vi "Manuele override - backup voor overbelasting.vi"() -> ()   [LabVIEW 2019]
panel:
  out "richtingsaanwijzer":dbl(knob) scale=0.0..10.0
  in  "kruispunt":string
  out "bericht":string
  in  "STOP":bool
  in  "START":bool
  in  "stop 2":bool
  out "address":u32
  out "port":u16
  in  "stop":bool
  in  "vooruit":bool
  in  "achteruit":bool
  in  "links":bool
  in  "rechts":bool
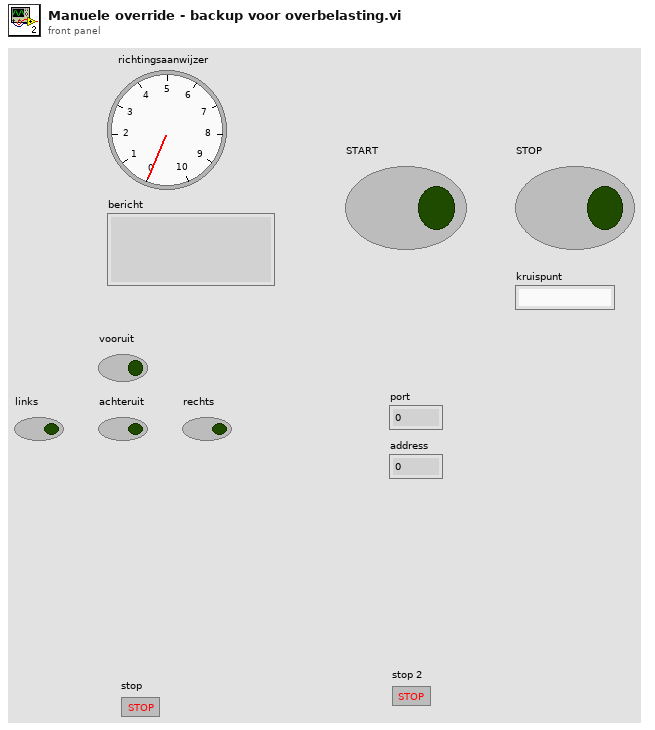
[diagram p1: front panel]
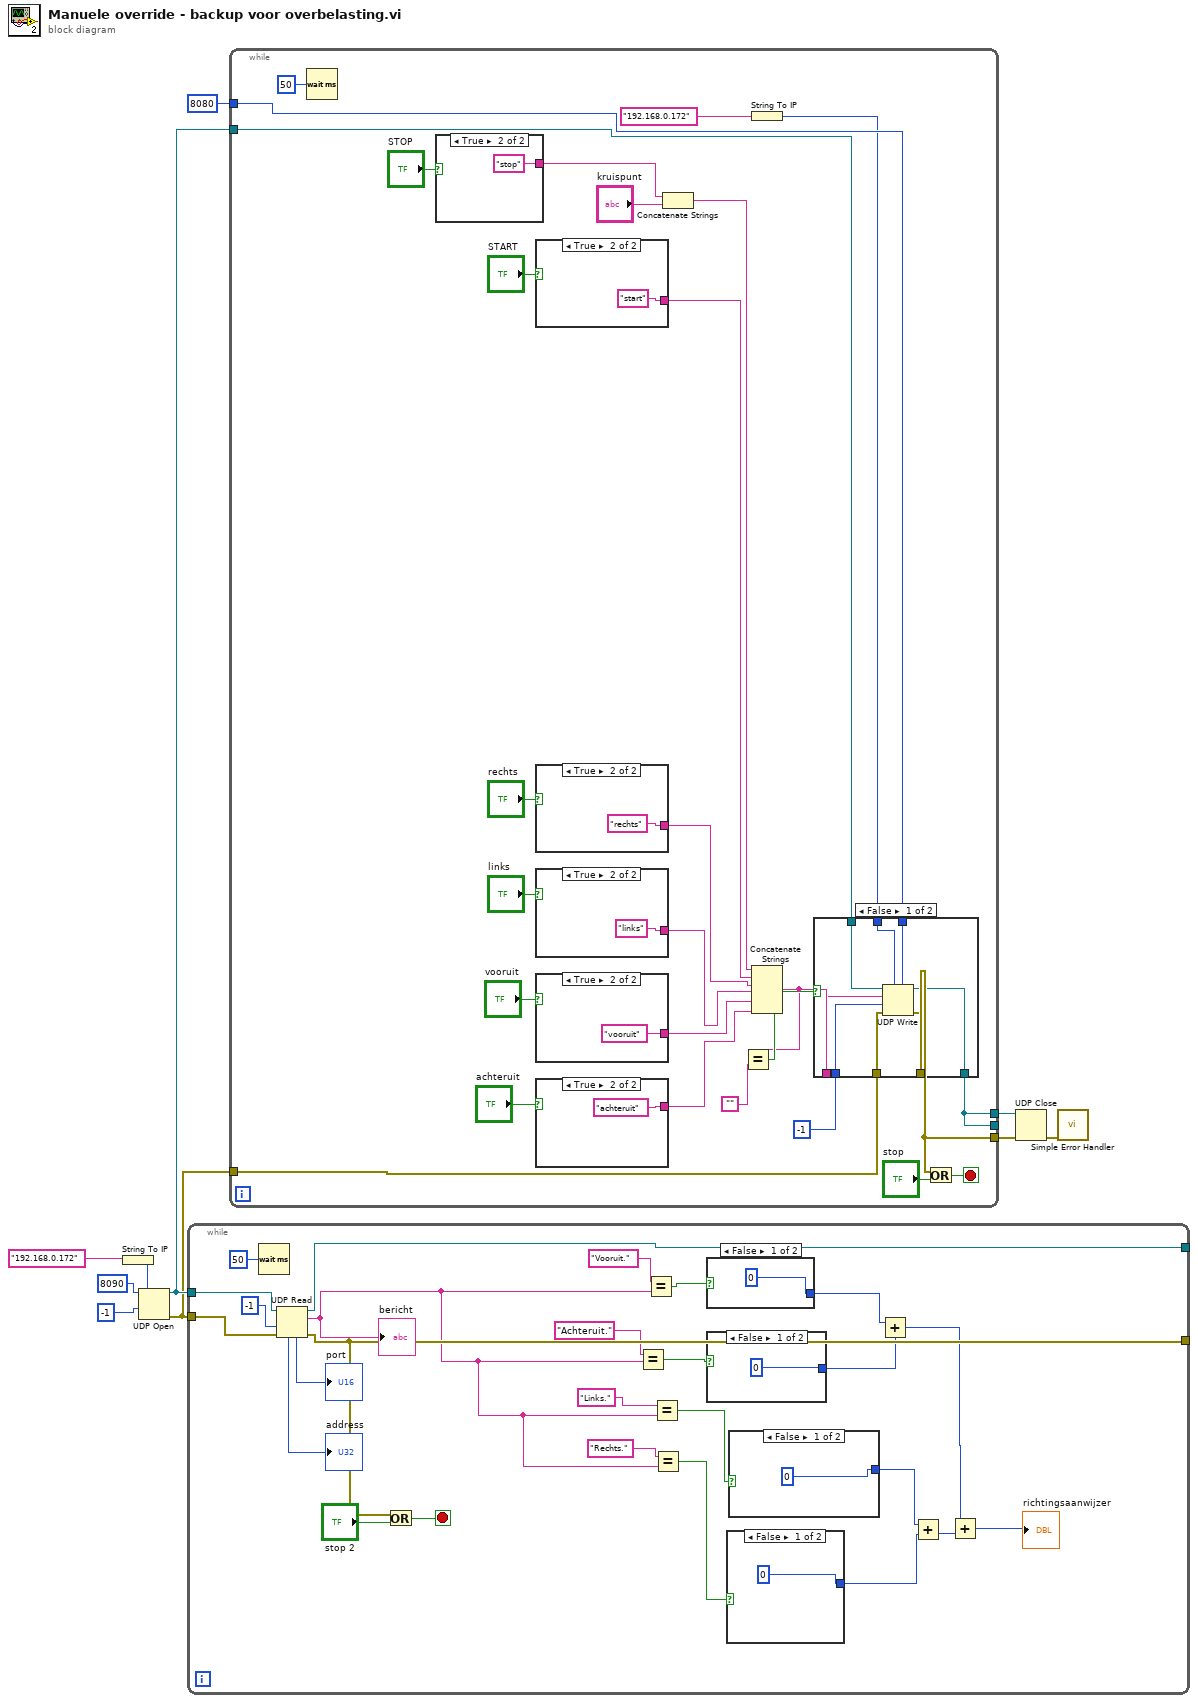
[diagram p0: block diagram]
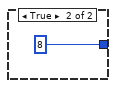
[diagram p2: hidden frame]
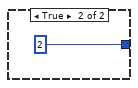
[diagram p3: hidden frame]
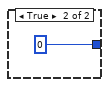
[diagram p4: hidden frame]
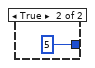
[diagram p5: hidden frame]
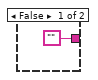
[diagram p7: hidden frame]
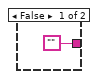
[diagram p8: hidden frame]
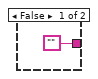
[diagram p9: hidden frame]
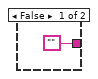
[diagram p10: hidden frame]
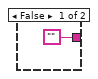
[diagram p11: hidden frame]
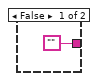
[diagram p12: hidden frame]
diagram:
  n1 = String To IP(1:"192.168.0.172") -> (0:w1:u32)
  n2 = UDP Open(7:w1, 9:-1, 11:8090) -> (port=w6:refnum<k16>, 0:w5:errorcluster)  [unwired: 2 in, 1 out]
  n3 = while {
    tunnel: w6 -> [w36]
    tunnel: w5 -> [w35]
    tunnel: [w32] -> _
    tunnel: [w31] -> _
    stop <- w29 stop-if-true
    n4 = Wait (ms)(milliseconds to wait=u32 50) -> ()  [unwired: 1 out]
    n5 = UDP Read(connection ID=w36, timeout ms (25000)=-1, 8:w35) -> (data out=w21:string, error out=w31:errorcluster, 3:w32:refnum<k16>, 4:→"port":u16, 6:→"address":u32)  [unwired: 1 in]
    "bericht" <- w21
    n6 = Or(x=w31, y="stop 2") -> (x .or. y?=w29:bool)
    n7 = Equal?(x="Achteruit.", y=w21) -> (x = y?=w20:bool)
    n8 = Equal?(x="Vooruit.", y=w21) -> (x = y?=w26:bool)
    n9 = Equal?(x="Links.", y=w21) -> (x = y?=w19:bool)
    n10 = Equal?(x="Rechts.", y=w21) -> (x = y?=w18:bool)
    n11 = case shown="False" w26 {
      tunnel: [0 5] -> w16
      frame False {
      }
      frame True {
      }
    }
    n12 = case shown="False" w20 {
      tunnel: [0 0] -> w17
      frame False {
      }
      frame True {
      }
    }
    n13 = case shown="False" w18 {
      tunnel: [0 8] -> w14
      frame False {
      }
      frame True {
      }
    }
    n14 = case shown="False" w19 {
      tunnel: [0 2] -> w15
      frame False {
      }
      frame True {
      }
    }
    n15 = Add(x=w16, y=w17) -> (x+y=w13:i32)
    n16 = Add(x=w15, y=w14) -> (x+y=w12:i32)
    n17 = Add(x=w13, y=w12) -> (x+y=→"richtingsaanwijzer":i32)
  }
  n18 = while {
    tunnel: w6 -> [w47]
    tunnel: w5 -> [w50]
    tunnel: 8080 -> [w52]
    tunnel: [w45] -> w4
    tunnel: [w46] -> w8
    tunnel: [w45] -> _
    stop <- w71 stop-if-true
    n19 = Wait (ms)(milliseconds to wait=50) -> ()  [unwired: 1 out]
    n20 = case shown="True" "STOP" {
      tunnel: ["" "stop"] -> w60
      frame False {
      }
      frame True {
      }
    }
    n21 = case shown="True" "START" {
      tunnel: ["" "start"] -> w64
      frame False {
      }
      frame True {
      }
    }
    n22 = case shown="True" "rechts" {
      tunnel: ["" "rechts"] -> w58
      frame False {
      }
      frame True {
      }
    }
    n23 = case shown="True" "links" {
      tunnel: ["" "links"] -> w57
      frame False {
      }
      frame True {
      }
    }
    n24 = case shown="True" "vooruit" {
      tunnel: ["" "vooruit"] -> w56
      frame False {
      }
      frame True {
      }
    }
    n25 = case shown="True" "achteruit" {
      tunnel: ["" "achteruit"] -> w55
      frame False {
      }
      frame True {
      }
    }
    n26 = Concatenate Strings(w60, "kruispunt") -> (w61:string)
    n27 = String To IP(1:"192.168.0.172") -> (0:w51:u32)
    n28 = Concatenate Strings(w61, w64, w58, w57, w56, w55) -> (w48:string)
    n29 = Equal?(x=w48, y="") -> (x = y?=w53:bool)
    n30 = case shown="False" w53 {
      tunnel: w52 -> [w80 _]
      tunnel: w51 -> [w79 _]
      tunnel: w50 -> [w78 w82]
      tunnel: -1 -> [w77 _]
      tunnel: w48 -> [w76 _]
      tunnel: w47 -> [w75 w81]
      tunnel: [w74 w82] -> w46
      tunnel: [w73 w81] -> w45
      frame False {
        n31 = UDP Write(address=w79, port or service name=w80, connection ID=w75, data in=w76, 8:w78, 9:w77) -> (error out=w74:errorcluster, 3:w73:refnum<k16>)
      }
      frame True {
      }
    }
    n32 = Or(x=w46, y="stop") -> (x .or. y?=w71:bool)
  }
  n33 = UDP Close(connection ID=w4, 8:w8) -> (error out=w7:errorcluster)  [unwired: 1 out]
  n34 = call <vilib>:"Simple Error Handler.vi"("error in (no error)"=w7) -> ()  [unwired: 4 in, 5 out]
